vi "TTS-MP3_POST.vi"() -> ()   [LabVIEW 2013]
uses:
  <vilib>/httpClient/POSTBuffer.vi
  <vilib>/httpClient/LabVIEWHTTPClient.lvlib
panel:
  in  "CN?":bool
  out "Numeric":i32
  in  "Loops":i32=1000
  in  "POST":bool
  out "ok?":bool
  in  "TEXT(UTF-8)":string
  in  "user":string="charles"
  out "error out":errorcluster
  out "body":string
  out "headers":string
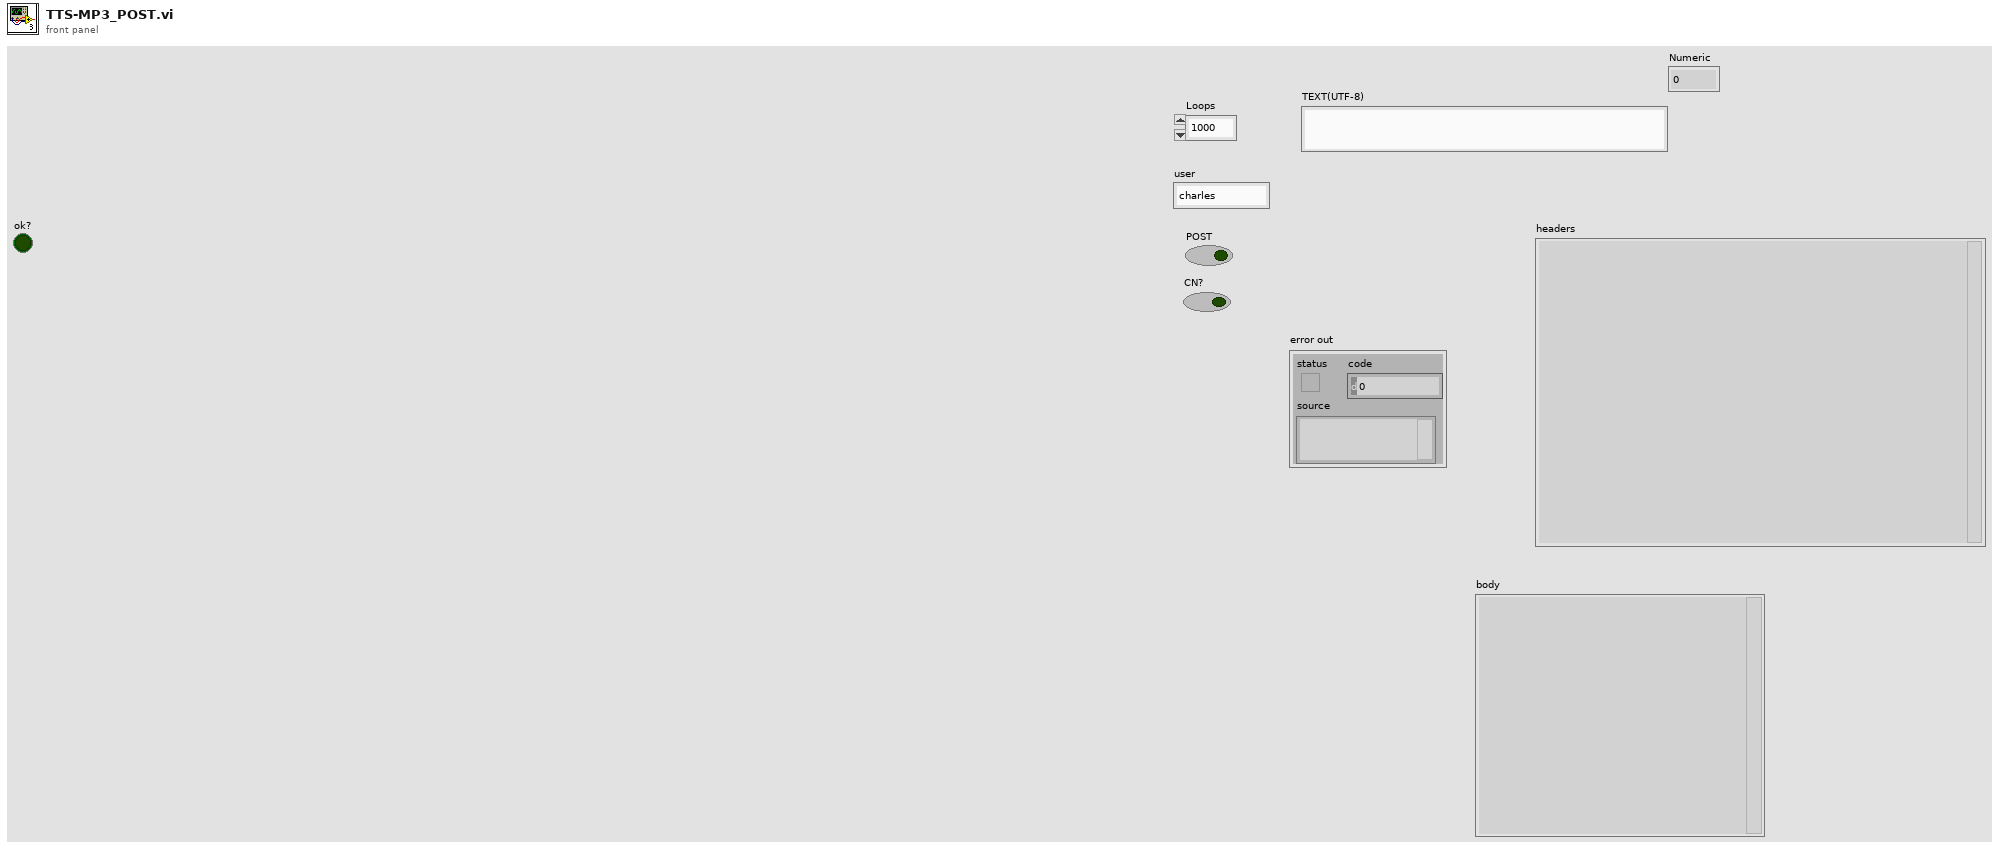
[diagram p1: front panel]
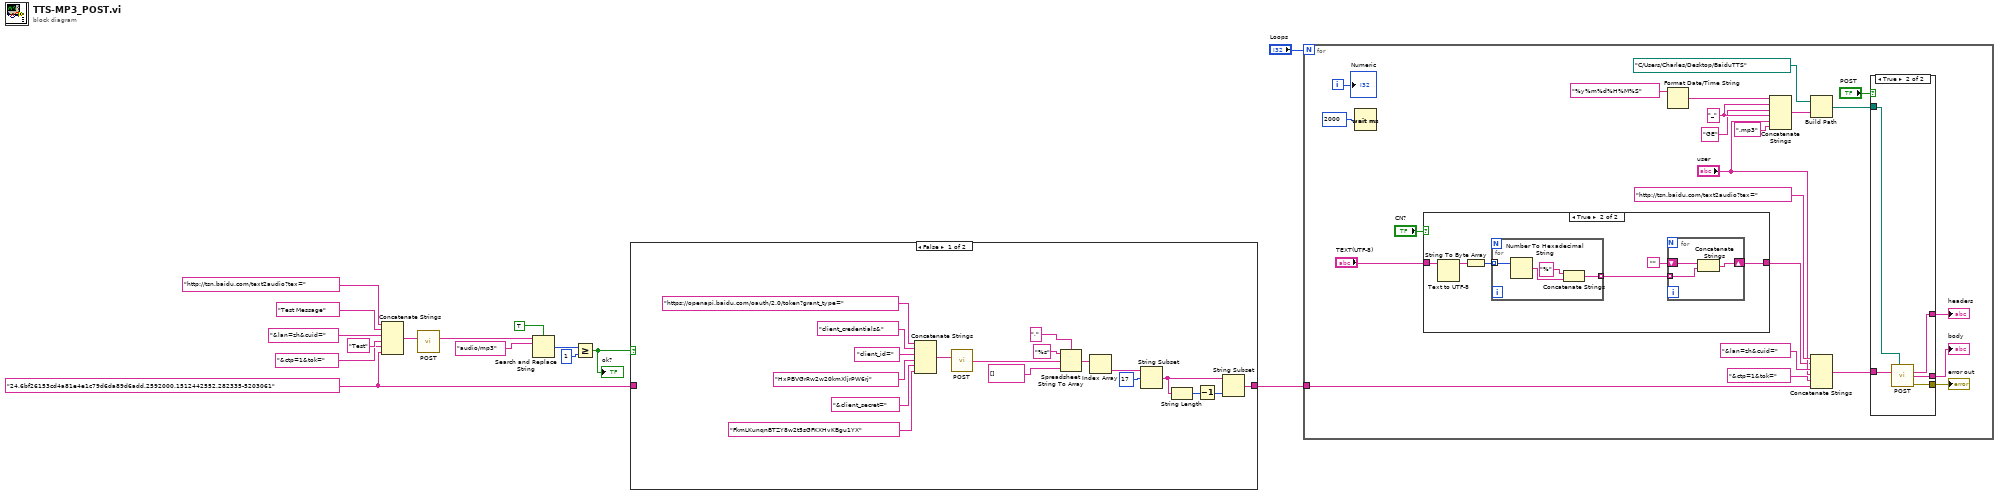
[diagram p0: block diagram]
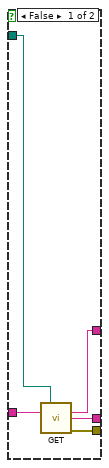
[diagram p3: hidden frame]
diagram:
  w3 = "24.6bf26153cd4a81e4e1c79d6da89d6add.2592000.1512442552.282335-5203061" ("Tok 2")
  n1 = Concatenate Strings("http://tsn.baidu.com/text2audio?tex=" ("string"), "Test Message" ("TEXT(UTF-8) 2"), "&lan=zh&cuid=" ("string"), "Test" ("user 2"), "&ctp=1&tok=" ("string"), w3) -> (w12:string)
  n2 = call-poly <vilib>:"POST.vi"("url"=w12) -> ("headers"=w5:string)  [unwired: 11 in, 3 out]
  n3 = Search and Replace String(case sensitive?=TRUE ("ignore case? (F)"), input string=w5, search string="audio/mp3") -> (number of replacements=w7:i32)  [unwired: 5 in, 3 out]
  n4 = Greater Or Equal?(x=w7, y=1) -> (x >= y?=w4:bool)
  "ok?" <- w4
  n5 = case shown="False" w4 {
    tunnel: w3 -> [_ w34]
    tunnel: [w16 w34] -> w2
    frame False {
      n6 = Concatenate Strings("https://openapi.baidu.com/oauth/2.0/token?grant_type=" ("string"), "client_credentials&" ("string"), "client_id=" ("string"), "HxPBVGrRw2w20kmXljrPW6rj" ("string"), "&client_secret=" ("string"), "FkmLKunqnBTZY8w2t5sGFKXHvKBgu1YX" ("string")) -> (w33:string)
      n7 = call-poly <vilib>:"POST.vi"("url"=w33) -> ("body"=w17:string)  [unwired: 11 in, 3 out]
      n8 = Spreadsheet String To Array(delimiter (Tab)=",", format string="%s", spreadsheet string=w17, array type (2D Dbl)=string[] []) -> (array=w23:string[])
      n9 = Index Array(array=w23) -> (element=w22:string)  [unwired: 1 in]
      n10 = String Subset(string=w22, offset (0)=17) -> (substring=w20:string)  [unwired: 1 in]
      n11 = String Length(string=w20) -> (length=w19:i32)
      n12 = Decrement(x=w19) -> (x-1=w18:i32)
      n13 = String Subset(string=w20, length (rest)=w18) -> (substring=w16:string)  [unwired: 1 in]
    }
    frame True {
    }
  }
  n14 = for {
    N: "Loops" -> [_]
    tunnel: w2 -> [w52]
    i -> [w38]
    w46 = "_" ("string")
    n15 = Wait (ms)(milliseconds to wait=u32 2000) -> ()  [unwired: 1 out]
    n16 = case shown="True" "CN?" {
      tunnel: [w58 w60] -> w37
      tunnel: "TEXT(UTF-8)" -> [w58 w59]
      frame False {
      }
      frame True {
        n17 = Text to UTF-8(11:w59) -> (3:w64:string)  [unwired: 1 in, 1 out]
        n18 = String To Byte Array(string=w64) -> (unsigned byte array=w63:u8[])
        n19 = for {
          tunnel: w63 -> [w71] mode=indexing
          tunnel: [w68] -> w62 mode=indexing
          n20 = Number To Hexadecimal String(2:w71) -> (0:w70:string)  [unwired: 1 in]
          n21 = Concatenate Strings("%" ("string"), w70) -> (w68:string)
        }
        n22 = for {
          tunnel: w62 -> [w65] mode=indexing
          shift-right: [w67] -> w60
          shift-left: "" -> [w66]
          n23 = Concatenate Strings(w66, w65) -> (w67:string)
        }
      }
    }
    n24 = Format Date/Time String(time format string (%c)="%y%m%d%H%M%S") -> (date/time string=w44:string)  [unwired: 2 in]
    n25 = Concatenate Strings(w44, w46, "GE" ("string"), w46, "user", ".mp3" ("string")) -> (w49:string)
    n26 = Build Path(base path=path "C:/Users/Charles/Desktop/BaiduTTS" ("file (use dialog)"), name or relative path=w49) -> (appended path=w50:path)
    n27 = Concatenate Strings("http://tsn.baidu.com/text2audio?tex=" ("string"), w37, "&lan=zh&cuid=" ("string"), "user", "&ctp=1&tok=" ("string"), w52) -> (w55:string)
    n28 = case shown="True" "POST" {
      tunnel: w55 -> [w75 w81]
      tunnel: [w74 w80] -> w53
      tunnel: w50 -> [w76 w79]
      tunnel: [w73 w78] -> w42
      tunnel: [w72 w77] -> w41
      frame False {
        n29 = call <vilib>:"GET.vi"("output file"=w76, "url"=w75) -> ("headers"=w73:string, "body"=w72:string, "error out"=w74:errorcluster)  [unwired: 10 in, 1 out]
      }
      frame True {
        n30 = call-poly <vilib>:"POST.vi"("output file"=w79, "url"=w81) -> ("headers"=w78:string, "body"=w77:string, "error out"=w80:errorcluster)  [unwired: 10 in, 1 out]
      }
    }
    "error out" <- w53
    "headers" <- w42
    "body" <- w41
    "Numeric" <- w38
  }
